vi "Configure Units.vi"(8 "error in":errorcluster, 11 "PRM in":refnum<class "PRM.lvclass">) -> (0 "error out":errorcluster, 3 "PRM out":refnum<class "PRM.lvclass">)   [LabVIEW 2019, in "PRM.lvlib" / "PRM.lvclass"]
uses:
  Library/PRM.lvclass
  Custom Controls/Units.ctl
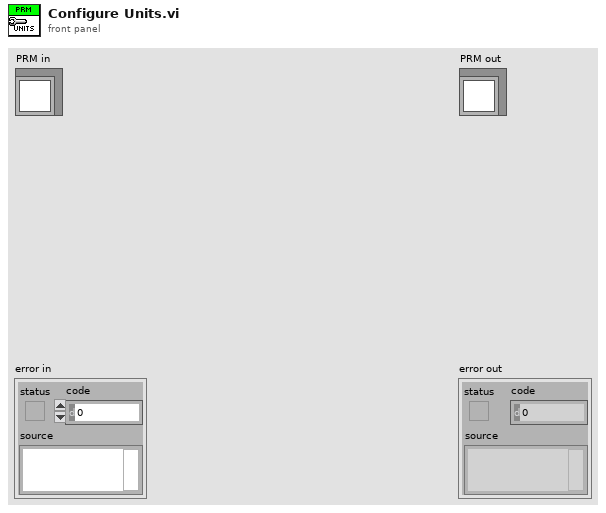
[diagram p1: front panel]
types:
  T1 = typedef "PRM.lvlib/PRM.lvclass/Units.ctl" = enum16{"Celsius", "Fahrenheit", "Kelvin", "Ohms"}
  T2 = typedef "PRM.lvlib/PRM.lvclass/Operational Mode.ctl" = enum16{"RESISTANCE", "TEMPERATURE", "POTENTIOMETER"}
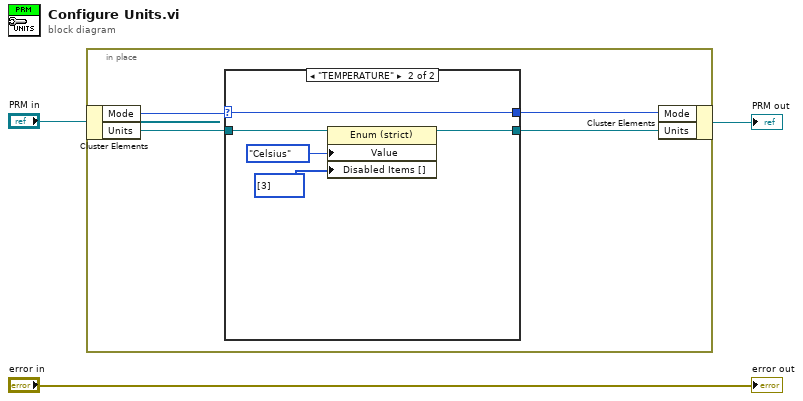
[diagram p0: block diagram]
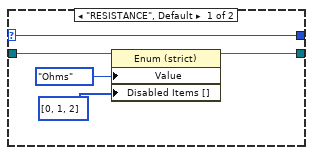
[diagram p2: hidden frame]
diagram:
  n1 = in-place {
    n2 = in-place-cluster #1("PRM in") -> ("Mode"=w7:T2, "Units"=w5:refnum<vi>)
    n3 = case shown="\"TEMPERATURE\"" w7 {
      selector: w7 -> [w12 w17]
      tunnel: [w12 w17] -> w6
      tunnel: w5 -> [w11 w16]
      tunnel: [w10 w15] -> w4
      frame "RESISTANCE", Default {
        n4 = property class="Enum (strict)"(reference=w11, "Value"=Units."Ohms", "Disabled Items []"=i32[] [0, 1, 2]) -> (reference out=w10:refnum<vi>)  [unwired: 1 in, 1 out]
      }
      frame "TEMPERATURE" {
        n5 = property class="Enum (strict)"(reference=w16, "Value"=Units."Celsius", "Disabled Items []"=i32[] [3]) -> (reference out=w15:refnum<vi>)  [unwired: 1 in, 1 out]
      }
    }
    n6 = in-place-cluster #1("Mode"=w6, "Units"=w4) -> (→"PRM out":refnum<class "PRM.lvclass">)
  }
  "error out" <- "error in"
